vi "Jog XY go_o.vi"(9 "Speed":dbl=5.0 format="%#_13g", 10 "Jog Cluster":T1={"Jog XY Cluster"={"object goes up"=FALSE, "object goes down"=FALSE, "object goes right"=FALSE, "object goes left"=FALSE, "SW2"=FALSE, "SW1"=FALSE, "YY (mm)"=0.1, "YN (mm) "=0.01, "NY (mm) "=0.005, "NN (mm) "=0.001}, "Jog Z Cluster "={"Z go down 0.1 mm"=FALSE, "Z go up 0.1 mm"=FALSE, "Z go down 0.05 mm"=FALSE, "Z go up 0.05 mm"=FALSE, "Z go down 0.01 mm"=FALSE, "Z go up 0.01 mm"=FALSE, "Z go down"=FALSE, "Z go up"=FALSE, "step (mm)"=0.001}}, 11 "A3200.lvclass IN":refnum<class "A3200.lvclass">) -> (2 "Jog Cluster output":T1={"Jog XY Cluster"={"object goes up"=FALSE, "object goes down"=FALSE, "object goes right"=FALSE, "object goes left"=FALSE, "SW2"=FALSE, "SW1"=FALSE, "YY (mm)"=0.1, "YN (mm) "=0.01, "NY (mm) "=0.005, "NN (mm) "=0.001}, "Jog Z Cluster "={"Z go down 0.1 mm"=FALSE, "Z go up 0.1 mm"=FALSE, "Z go down 0.05 mm"=FALSE, "Z go up 0.05 mm"=FALSE, "Z go down 0.01 mm"=FALSE, "Z go up 0.01 mm"=FALSE, "Z go down"=FALSE, "Z go up"=FALSE, "step (mm)"=0.001}}, 3 "A3200.lvclass OUT":refnum<class "A3200.lvclass">)   [LabVIEW 2016]
uses:
  Classes/Controller/Motion/A3200 Folder/A3200.lvclass
panel:
  in  "Tab Control":enum32{"jog", "controller"}(tab)
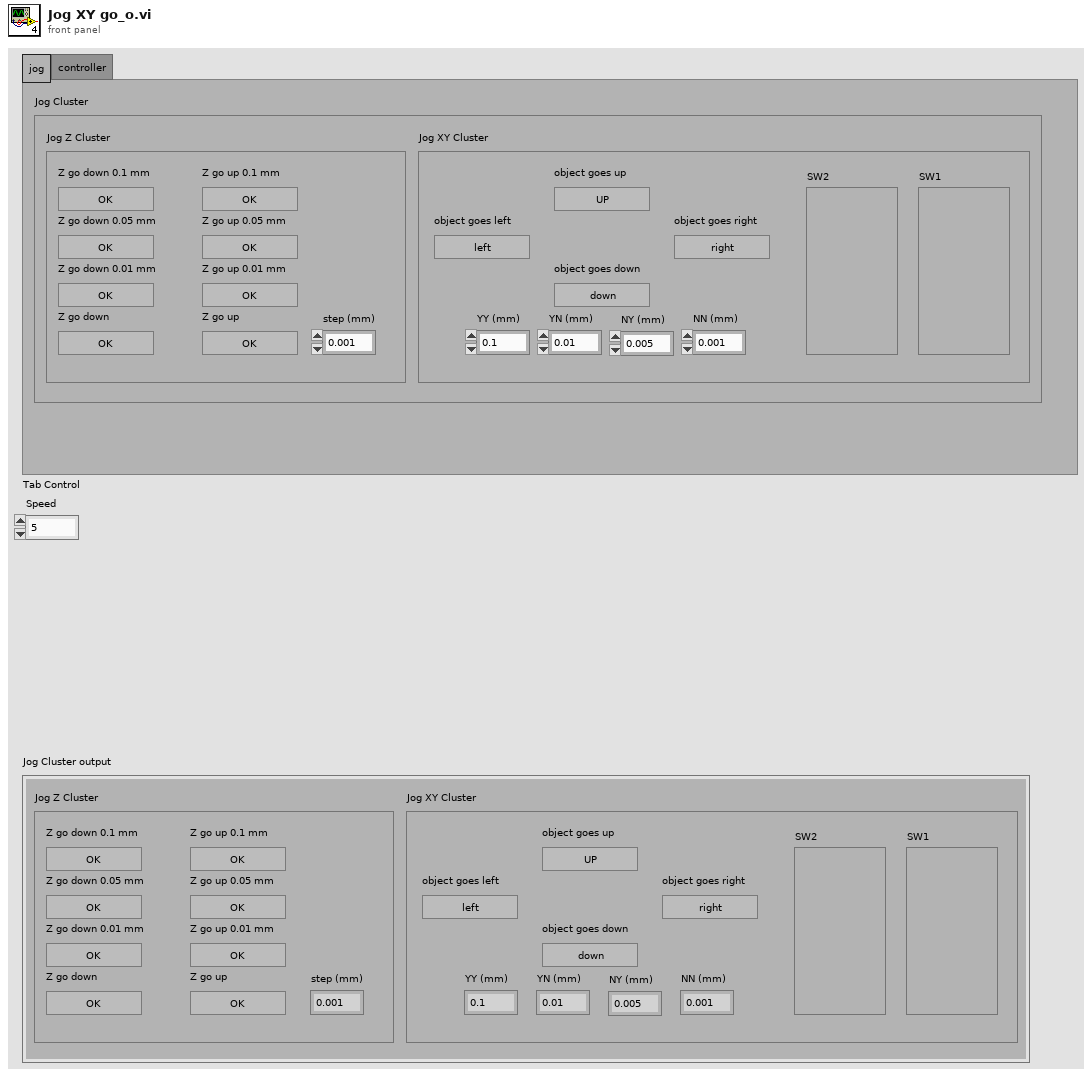
[diagram p1: front panel]
types:
  T1 = cluster{"Jog XY Cluster":cluster{"object goes up":bool, "object goes down":bool, "object goes right":bool, "object goes left":bool, "SW2":bool, "SW1":bool, "YY (mm)":dbl, "YN (mm) ":dbl, "NY (mm) ":dbl, "NN (mm) ":dbl}, "Jog Z Cluster ":cluster{"Z go down 0.1 mm":bool, "Z go up 0.1 mm":bool, "Z go down 0.05 mm":bool, "Z go up 0.05 mm":bool, "Z go down 0.01 mm":bool, "Z go up 0.01 mm":bool, "Z go down":bool, "Z go up":bool, "step (mm)":dbl}}
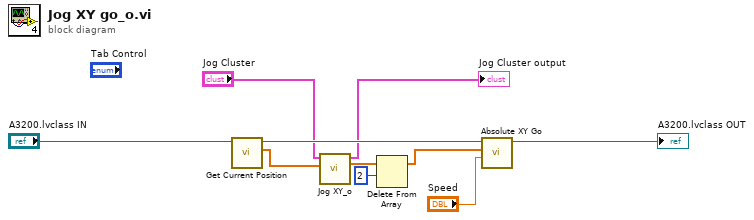
[diagram p0: block diagram]
diagram:
  n1 = call-dynamic "Get Current Position.vi"("Gantry in"="A3200.lvclass IN") -> ("XYZTheta Out"=w8:dbl[], "Gantry out"=w5:refnum<class "A3200.lvclass">)  [unwired: 8 in, 1 out]
  n2 = call "Jog XY_o.vi"("array IN"=w8, "Jog Cluster"="Jog Cluster") -> ("array OUT"=w10:dbl[], "Jog Cluster 2"=→"Jog Cluster output":T1)  [unwired: 8 in]
  n3 = Delete From Array(array=w10, length=2) -> (array with subset deleted=w3:dbl[])  [unwired: 1 in, 1 out]
  n4 = call-dynamic "Absolute XY Go.vi"("Speed"="Speed", "XY"=w3, "Gantry in"=w5) -> ("Gantry out"=→"A3200.lvclass OUT":refnum<class "A3200.lvclass">)  [unwired: 7 in, 1 out]
